vi "Keithley 6221 Sweep.vi"() -> ()   [LabVIEW 2024]
panel:
  in  "stop":bool
  in  "Log Sweep?":bool
  in  "Compliance Voltage":dbl format="%.3f"
  in  "Sweep Time (H:M:S)":dbl format="%<%H:%M:%S>t"
  in  "Stop Current":dbl=0.007 min=-0.007 max=0.007 format="%^.3e"
  in  "Start Current":dbl min=-0.105 max=0.007 format="%^.3e"
  in  "Output Off":bool
  in  "Start Sweep":bool
  in  "Setup":bool
  in  "VISA resource name":refnum<visa-resource-name>
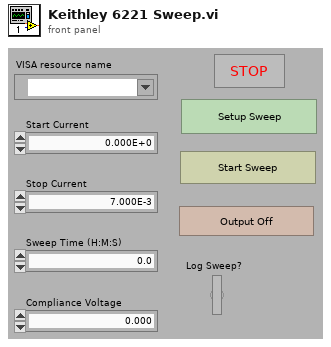
[diagram p1: front panel]
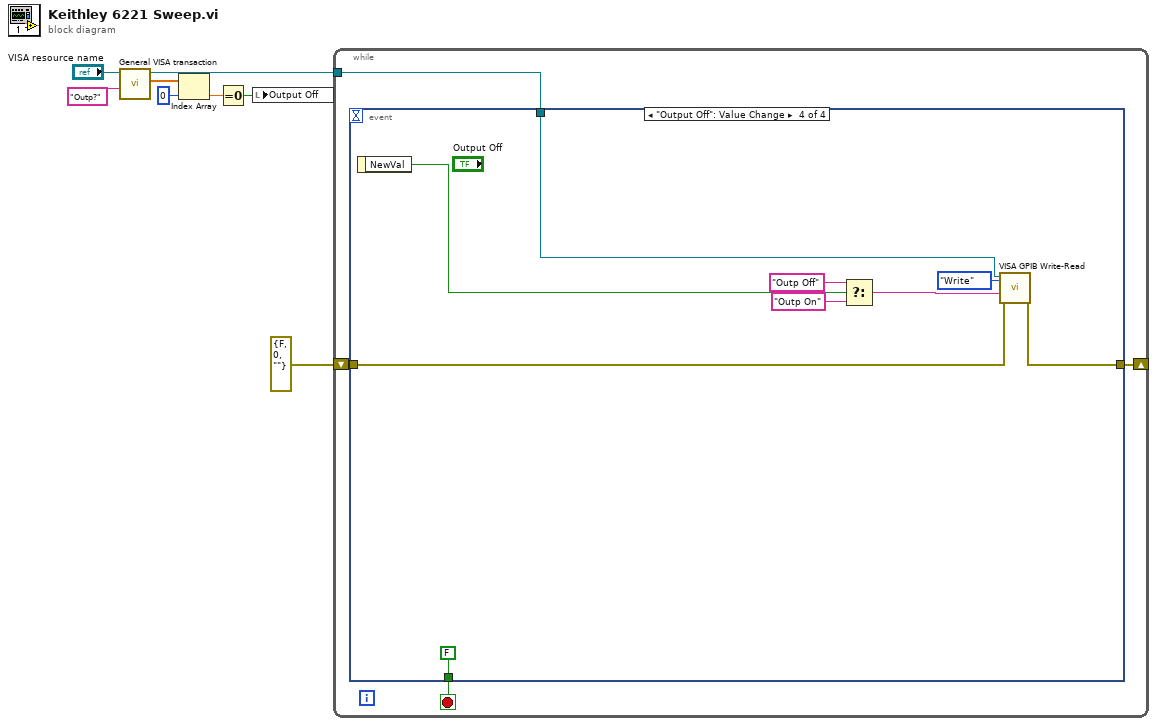
[diagram p0: block diagram]
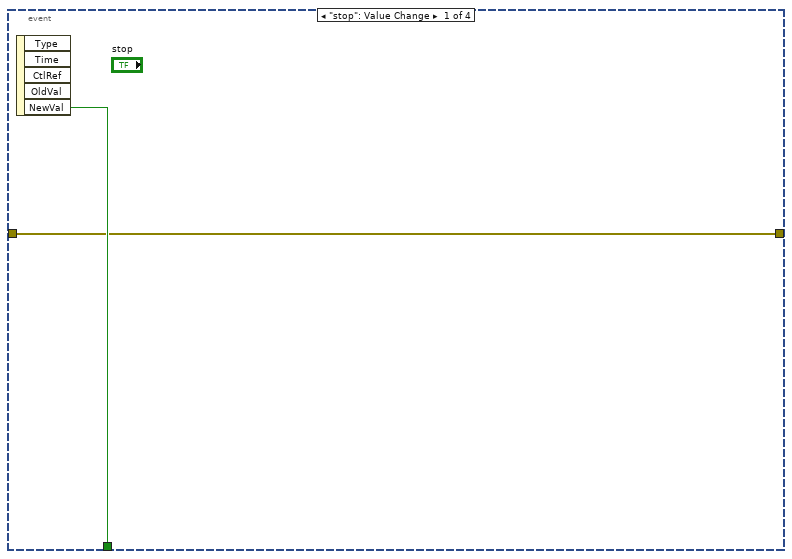
[diagram p2: hidden frame]
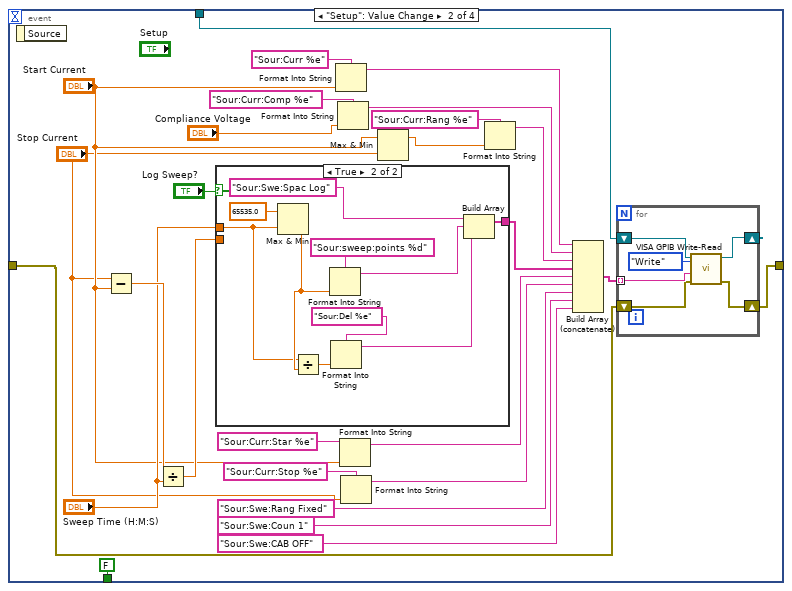
[diagram p3: hidden frame]
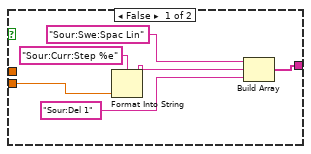
[diagram p4: hidden frame]
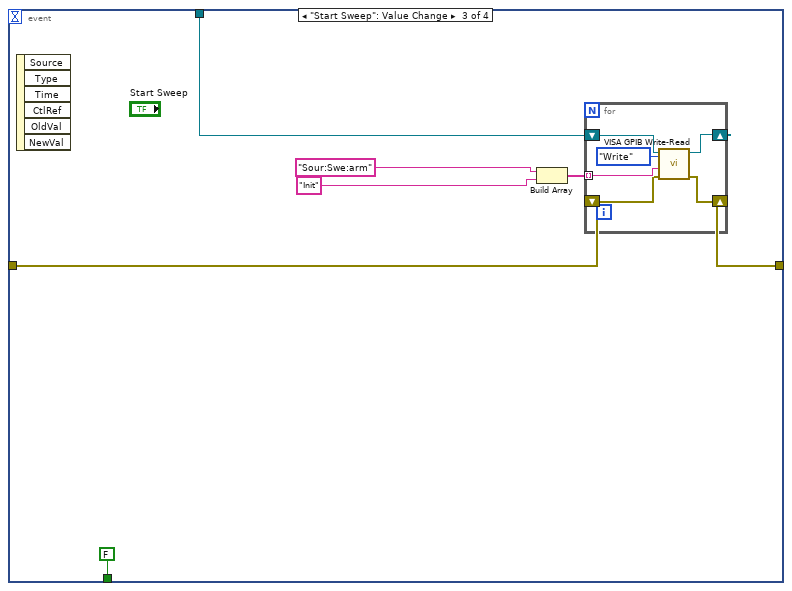
[diagram p5: hidden frame]
diagram:
  n1 = call "General VISA transaction.vi"("Command String"="Outp?" ("String to Write"), "VISA Session"="VISA resource name") -> ("Measurement"=w4:dbl[], "dup VISA Session"=w6:refnum<visa-resource-name>)  [unwired: 4 in, 4 out]
  n2 = Index Array(array=w4, index=0) -> (element=w2:dbl)
  n3 = Equal To 0?(x=w2) -> (x = 0?=w1:bool)
  n4 = local write "Output Off"(w1) -> ()
  n5 = while {
    shift-right: [w11] -> _
    shift-left: errorcluster {"status"=FALSE, "code"=0, "source"=""} ("error out") -> [w10]
    tunnel: w6 -> [w9]
    stop <- w12 stop-if-true
    n6 = event shown="[3] \"Output Off\": Value Change" {
      selector: _ -> [_ _ _ _]
      dyn-events: _ -> [_ _ _ _]
      timeout: _ -> [_ _ _ _]
      tunnel: w9 -> [_ w29 w70 w85]
      tunnel: [w14 FALSE ("NewVal") FALSE ("NewVal") FALSE ("NewVal")] -> w12
      tunnel: [w13 w26 w64 w82] -> w11
      tunnel: w10 -> [w13 w25 w65 w81]
      event "stop": Value Change {
        n7 = event-data() -> ("NewVal"=w14:bool)  [unwired: 1 in, 4 out]
      }
      event "Setup": Value Change {
        n8 = event-data() -> ()  [unwired: 1 in, 1 out]
        n9 = Subtract(x="Stop Current", y="Start Current") -> (x-y=w24:dbl)
        n10 = Divide(x=w24, y="Sweep Time (H:M:S)") -> (x/y=w22:dbl)
        n11 = case shown="True" "Log Sweep?" {
          tunnel: w22 -> [w46 _]
          tunnel: [w43 w57] -> w21
          tunnel: "Sweep Time (H:M:S)" -> [_ w48]
          frame False {
            n12 = Format Into String(format string="Sour:Curr:Step %e", w46) -> (resulting string=w45:string)  [unwired: 2 in, 1 out]
            n13 = Build Array("Sour:Swe:Spac Lin", w45, "Sour:Del 1") -> (w43:string[])
          }
          frame True {
            n14 = Max & Min(x=65535.0, y=w48) -> (min(x,y)=w49:dbl)  [unwired: 1 out]
            n15 = Divide(x=w48, y=w49) -> (x/y=w51:dbl)
            n16 = Format Into String(format string="Sour:sweep:points %d", w49) -> (resulting string=w53:string)  [unwired: 2 in, 1 out]
            n17 = Format Into String(format string="Sour:Del %e", w51) -> (resulting string=w50:string)  [unwired: 2 in, 1 out]
            n18 = Build Array("Sour:Swe:Spac Log", w53, w50) -> (w57:string[])
          }
        }
        n19 = Format Into String(format string="Sour:Curr %e", "Start Current") -> (resulting string=w37:string)  [unwired: 2 in, 1 out]
        n20 = Format Into String(format string="Sour:Curr:Comp %e", "Compliance Voltage") -> (resulting string=w36:string)  [unwired: 2 in, 1 out]
        n21 = Format Into String(format string="Sour:Curr:Star %e", "Start Current") -> (resulting string=w35:string)  [unwired: 2 in, 1 out]
        n22 = Format Into String(format string="Sour:Curr:Stop %e", "Stop Current") -> (resulting string=w34:string)  [unwired: 2 in, 1 out]
        n23 = Max & Min(x="Start Current", y="Stop Current") -> (max(x,y)=w18:dbl)  [unwired: 1 out]
        n24 = Format Into String(format string="Sour:Curr:Rang %e", w18) -> (resulting string=w15:string)  [unwired: 2 in, 1 out]
        n25 = Build Array (concatenate)(w37, w36, w15, w21, w35, w34, "Sour:Swe:Rang Fixed", "Sour:Swe:Coun 1", "Sour:Swe:CAB OFF") -> (w30:string[])
        n26 = for {
          tunnel: w30 -> [w62] mode=indexing
          shift-right: [w60] -> _
          shift-left: w29 -> [w61]
          shift-right: [w58] -> w26
          shift-left: w25 -> [w59]
          n27 = call "VISA GPIB Write-Read.vi"("error in (no error)"=w59, "Command"=w62, "Action"=enum16{"Write", "Read", "Write & Read"}."Write", "VISA resource name"=w61) -> ("error out"=w58:errorcluster, "dup VISA Session"=w60:refnum<visa-resource-name>)  [unwired: 4 in, 2 out]
        }
      }
      event "Start Sweep": Value Change {
        n28 = event-data() -> ()  [unwired: 1 in, 6 out]
        n29 = Build Array("Sour:Swe:arm", "Init") -> (w69:string[])
        n30 = for {
          tunnel: w69 -> [w75] mode=indexing
          shift-right: [w73] -> _
          shift-left: w70 -> [w74]
          shift-right: [w71] -> w64
          shift-left: w65 -> [w72]
          n31 = call "VISA GPIB Write-Read.vi"("error in (no error)"=w72, "Command"=w75, "Action"=enum16{"Write", "Read", "Write & Read"}."Write", "VISA resource name"=w74) -> ("error out"=w71:errorcluster, "dup VISA Session"=w73:refnum<visa-resource-name>)  [unwired: 4 in, 2 out]
        }
      }
      event "Output Off": Value Change {
        n32 = event-data() -> ("NewVal"=w77:bool)  [unwired: 1 in]
        n33 = Select(t="Outp Off", s=w77, f="Outp On") -> (s? t:f=w80:string)
        n34 = call "VISA GPIB Write-Read.vi"("error in (no error)"=w81, "Command"=w80, "Action"=enum16{"Write", "Read", "Write & Read"}."Write", "VISA resource name"=w85) -> ("error out"=w82:errorcluster)  [unwired: 4 in, 3 out]
      }
    }
  }
